vi "get_all_messeges_chronologically.vi"(10 "DIAGNOSTIC_buffer_all_info":T1[][](array[typedef]), 11 "circular_buffer_positions":i32[](array[numeric])) -> (3 "all_messages":T1[](array[typedef]))   [LabVIEW 2020]
uses:
  FGV/DIAGNOSTICS_message_history_buffer/PROXY_DIAGNOSTICS_message_history_buffer_all_info.ctl
  STATION/station.ctl
  _misc/DIAGNOSTICS_message_type.ctl
  <userlib>/_OpenG.lib/array/array.llb/Filter 1D Array with Scalar (Variant)__ogtk.vi
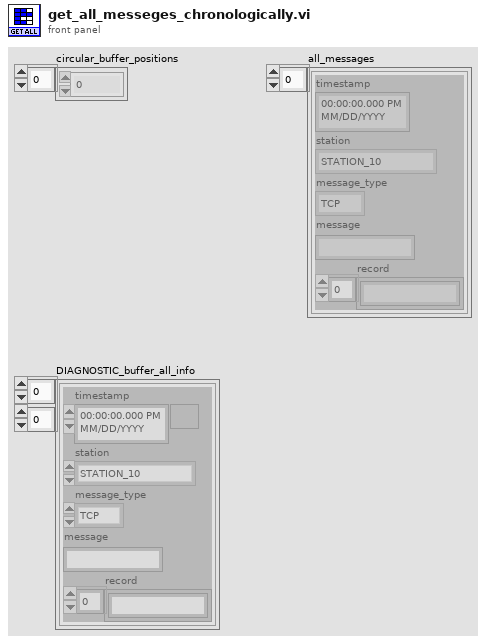
[diagram p1: front panel]
types:
  T1 = typedef "PROXY_DIAGNOSTICS_message_history_buffer_all_info.ctl" = cluster{"timestamp":timestamp, "station":T2, "message_type":T3, "message":string, "record":string[]}
  T2 = typedef "station.ctl" = enum16{"STATION_10", "STATION_20", "STATION_30", "STATION_40", "STATION_50", "STATION_60", "STATION_70", "STATION_80", "STATION_90", "STATION_100", "STATION_110", "STATION_120", "STATION_165", "MAIN"}
  T3 = typedef "DIAGNOSTICS_message_type.ctl" = enum16{"TCP", "SQL"}
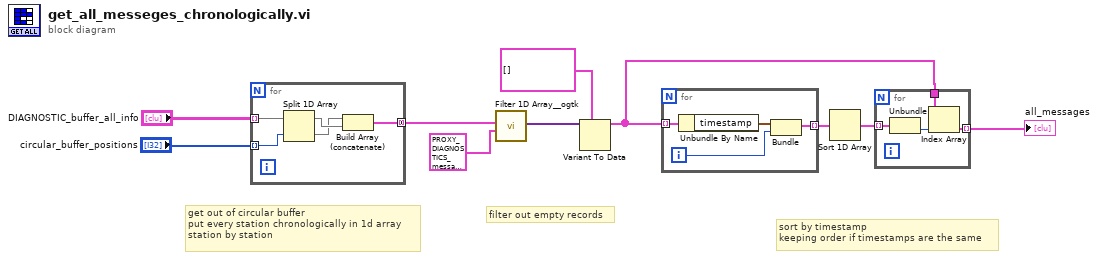
[diagram p0: block diagram]
diagram:
  # "sort by timestamp\nkeeping order if timestamps are the same"
  # "filter out empty records"
  # "get out of circular buffer\nput every station chronologically in 1d array\nstation by station"
  n1 = for {
    tunnel: "DIAGNOSTIC_buffer_all_info" -> [w13] mode=indexing
    tunnel: "circular_buffer_positions" -> [w12] mode=indexing
    tunnel: [w11] -> w6 mode=concatenating
    n2 = Split 1D Array(array=w13, index=w12) -> (first subarray=w15:T1[], second subarray=w14:T1[])
    n3 = Build Array (concatenate)(w14, w15) -> (w11:T1[])
  }
  n4 = call-poly <userlib>:"Filter 1D Array__ogtk.vi"("items to filter"=T1 {"timestamp"=timestamp(0 s since 1904-01-01), "station"=enum."STATION_10", "message_type"=enum."TCP", "message"="", "record"=[]} ("Cluster"), "array"=w6) -> ("filtered array"=w4:variant[])  [unwired: 4 in, 1 out]
  n5 = Variant To Data(type=T1[] [], Variant=w4) -> (data=w9:T1[])  [unwired: 1 in, 1 out]
  n6 = for {
    tunnel: w9 -> [w19] mode=indexing
    tunnel: [w16] -> w8 mode=indexing
    i -> [w17]
    n7 = Unbundle By Name(w19) -> ("timestamp"=w18:timestamp)
    n8 = Bundle("timestamp"=w18, w17) -> (w16:cluster{"timestamp":timestamp, i32})  [unwired: 1 in]
  }
  n9 = Sort 1D Array(array=w8) -> (sorted array=w7:cluster{"timestamp":timestamp, i32}[])
  n10 = for {
    tunnel: w7 -> [w23] mode=indexing
    tunnel: w9 -> [w21]
    tunnel: [w20] -> w10 mode=indexing
    n11 = Unbundle(w23) -> (w22:i32)  [unwired: 1 out]
    n12 = Index Array(array=w21, index=w22) -> (element=w20:T1)
  }
  "all_messages" <- w10
